vi "Numerical Integration.vi"(9 "Reset?":bool, 10 "dt":dbl, 11 "Data":dbl) -> (3 "Integrated Data":dbl format="%0.4f")   [LabVIEW 2023]
uses:
  <vilib>/Analysis/2dsp.llb/Integral Method.ctl
  <vilib>/Analysis/8numeric.llb/1D Numeric Integration.vi
  <vilib>/Analysis/NI_AALPro.lvlib
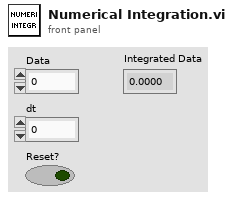
[diagram p1: front panel]
types:
  T1 = typedef "NI_AALPro.lvlib/Integral Method.ctl" = i32
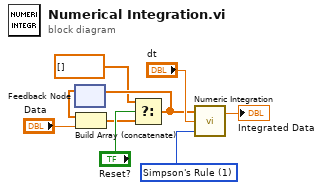
[diagram p0: block diagram]
diagram:
  w7 = T1 1 items=["Trapezoidal Rule", "Simpson's Rule", "Simpson's 3/8 Rule", "Bode Rule"] ("integration method")
  n1 = feedback #1() -> (w3:dbl[])  [unwired: 1 in]
  n2 = Build Array (concatenate)(w3, "Data") -> (w4:dbl[])
  n3 = Select(t=dbl[] [], s="Reset?", f=w4) -> (s? t:f=w8:dbl[])
  n4 = feedback-in #1(w8) -> ()
  n5 = call-poly <vilib>:"Numeric Integration.vi"("integration method"=w7, "dt"="dt", "Input Array"=w8) -> ("result"=→"Integrated Data":dbl)  [unwired: 1 out]
